vi "Generate Error.vi"(8 "Error In":errorcluster, 11 "DJTG Error":T1) -> (0 "Error Out":errorcluster)   [LabVIEW 2011, in "LVH-Adept.lvlib" / "DJTG.lvlib"]
uses:
  DJTG.lvlib
  Type Defs/Error.ctl
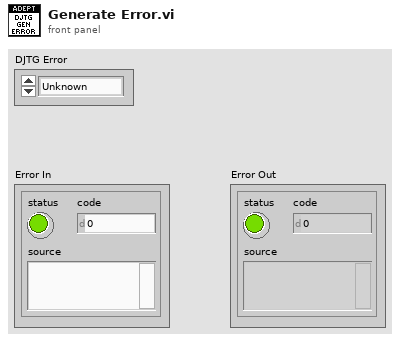
[diagram p1: front panel]
types:
  T1 = typedef "LVH-Adept.lvlib/DJTG.lvlib/Error.ctl" = enum16{"Unknown", "Enable", "PutTmsTdiBits", "GetTdoBits", "Disable", "Close", "Set Aux Reset", "Port Properties", "Get Speed", "Set Speed", "Get Port Count", "Get Batch Properties", "Enable Port", "Set Tmd Tdi Tck", "Get Tms Tdi Tdo Tck", "Put Tdi Bits", "Put Tms Bits", "Clock Tck", "Wait", "Batch"}
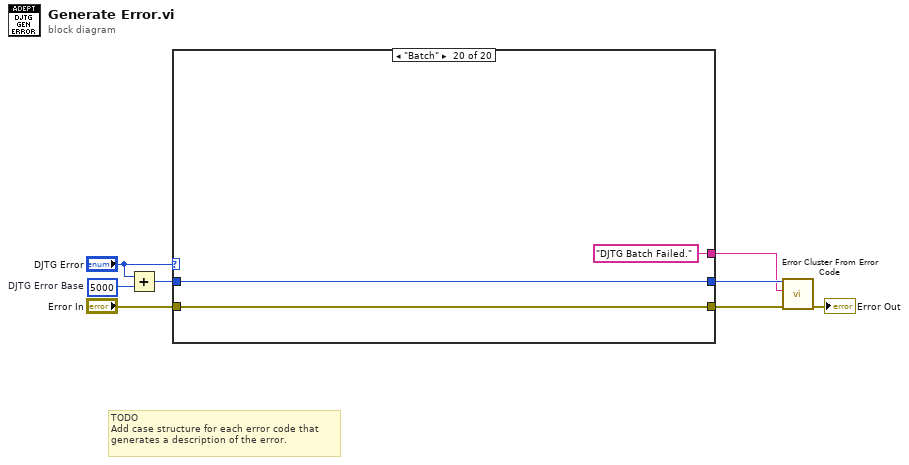
[diagram p0: block diagram]
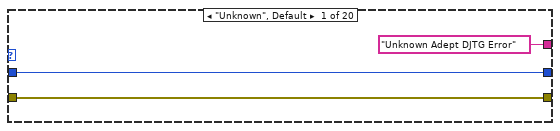
[diagram p2: hidden frame]
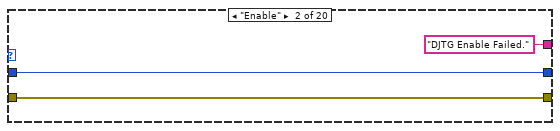
[diagram p3: hidden frame]
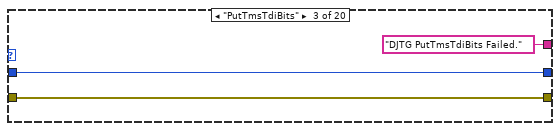
[diagram p4: hidden frame]
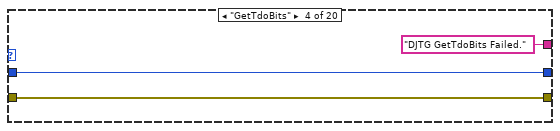
[diagram p5: hidden frame]
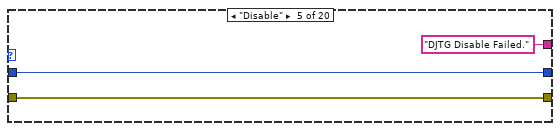
[diagram p6: hidden frame]
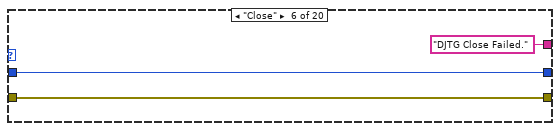
[diagram p7: hidden frame]
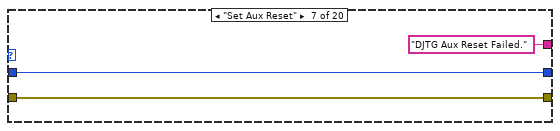
[diagram p8: hidden frame]
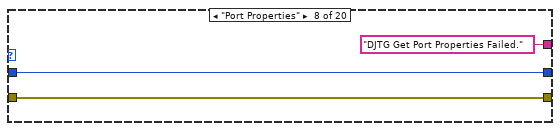
[diagram p9: hidden frame]
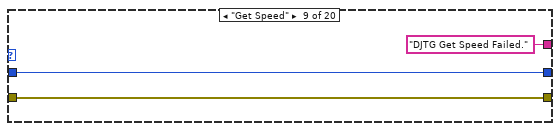
[diagram p10: hidden frame]
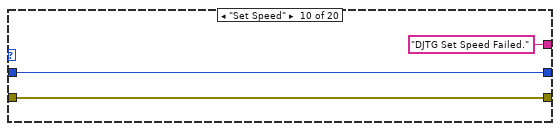
[diagram p11: hidden frame]
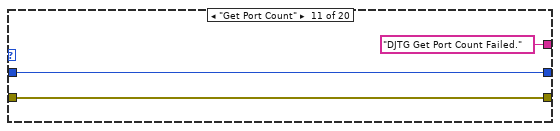
[diagram p12: hidden frame]
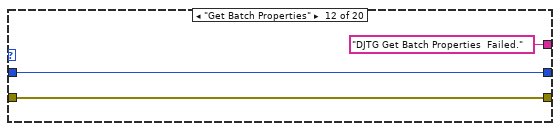
[diagram p13: hidden frame]
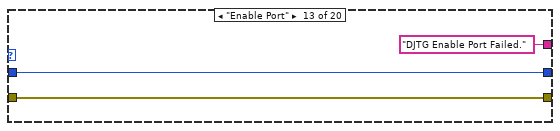
[diagram p14: hidden frame]
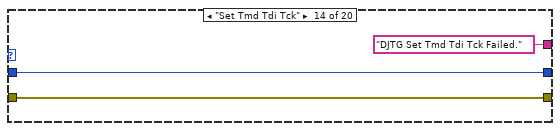
[diagram p15: hidden frame]
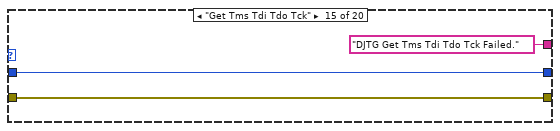
[diagram p16: hidden frame]
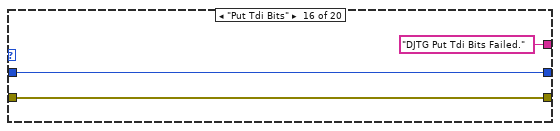
[diagram p17: hidden frame]
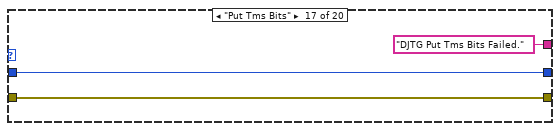
[diagram p18: hidden frame]
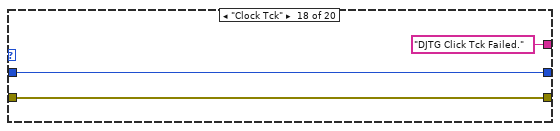
[diagram p19: hidden frame]
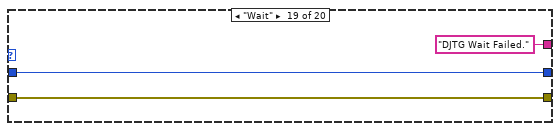
[diagram p20: hidden frame]
diagram:
  w5 = 5000  # DJTG Error Base
  # "TODO\nAdd case structure for each error code that \ngenerates a description of the error."
  n1 = Add(x="DJTG Error", y=w5) -> (x+y=w2:i32)
  n2 = case shown="\"Batch\"" "DJTG Error" {
    tunnel: [w11 w13 w16 w19 w22 w25 w28 w31 w34 w37 w40 w43 w46 w49 w52 w55 w58 w61 w64 w67] -> w7
    tunnel: "Error In" -> [w11 w13 w16 w19 w22 w25 w28 w31 w34 w37 w40 w43 w46 w49 w52 w55 w58 w61 w64 w67]
    tunnel: [w9 w14 w17 w20 w23 w26 w29 w32 w35 w38 w41 w44 w47 w50 w53 w56 w59 w62 w65 w68] -> w4
    tunnel: ["Unknown Adept DJTG Error" "DJTG Enable Failed." "DJTG PutTmsTdiBits Failed." "DJTG GetTdoBits Failed." "DJTG Disable Failed." "DJTG Close Failed." "DJTG Aux Reset Failed." "DJTG Get Port Properties Failed." "DJTG Get Speed Failed." "DJTG Set Speed Failed." "DJTG Get Port Count Failed." "DJTG Get Batch Properties  Failed." "DJTG Enable Port Failed." "DJTG Set Tmd Tdi Tck Failed." "DJTG Get Tms Tdi Tdo Tck Failed." "DJTG Put Tdi Bits Failed." "DJTG Put Tms Bits Failed." "DJTG Click Tck Failed." "DJTG Wait Failed." "DJTG Batch Failed."] -> w3
    tunnel: w2 -> [w9 w14 w17 w20 w23 w26 w29 w32 w35 w38 w41 w44 w47 w50 w53 w56 w59 w62 w65 w68]
    frame "Unknown", Default {
    }
    frame "Enable" {
    }
    frame "PutTmsTdiBits" {
    }
    frame "GetTdoBits" {
    }
    frame "Disable" {
    }
    frame "Close" {
    }
    frame "Set Aux Reset" {
    }
    frame "Port Properties" {
    }
    frame "Get Speed" {
    }
    frame "Set Speed" {
    }
    frame "Get Port Count" {
    }
    frame "Get Batch Properties" {
    }
    frame "Enable Port" {
    }
    frame "Set Tmd Tdi Tck" {
    }
    frame "Get Tms Tdi Tdo Tck" {
    }
    frame "Put Tdi Bits" {
    }
    frame "Put Tms Bits" {
    }
    frame "Clock Tck" {
    }
    frame "Wait" {
    }
    frame "Batch" {
    }
  }
  n3 = call <vilib>:"Error Cluster From Error Code.vi"("error in (no error)"=w7, "error message (\"\")"=w3, "error code (0)"=w4) -> ("error out"=→"Error Out":errorcluster)  [unwired: 6 in]
